vi "Sending Single U32 CMD and String Data.vi"(0 "TCP Ref In":refnum<k5>, 1 "Time Out(ms)":i32=100, 5 "CMD":u32, 9 "Data":string, 11 "error in (no error)":errorcluster) -> (4 "TCP Ref Out":refnum<k5>, 15 "error out":errorcluster)   [LabVIEW 2024]
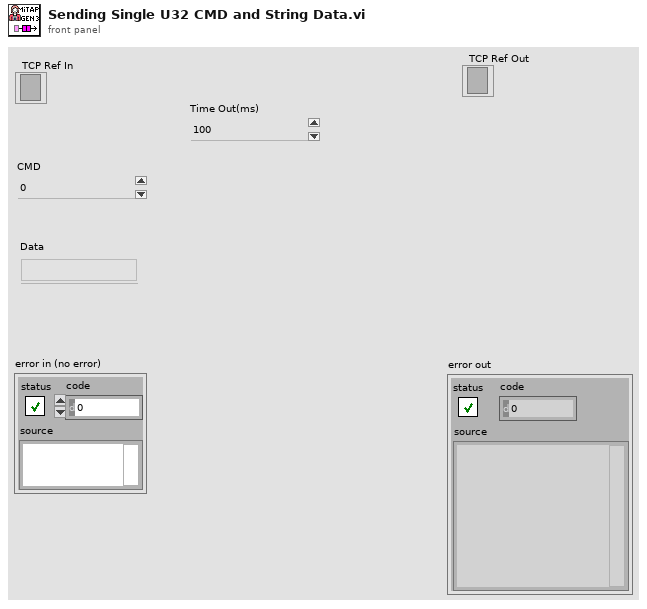
[diagram p1: front panel]
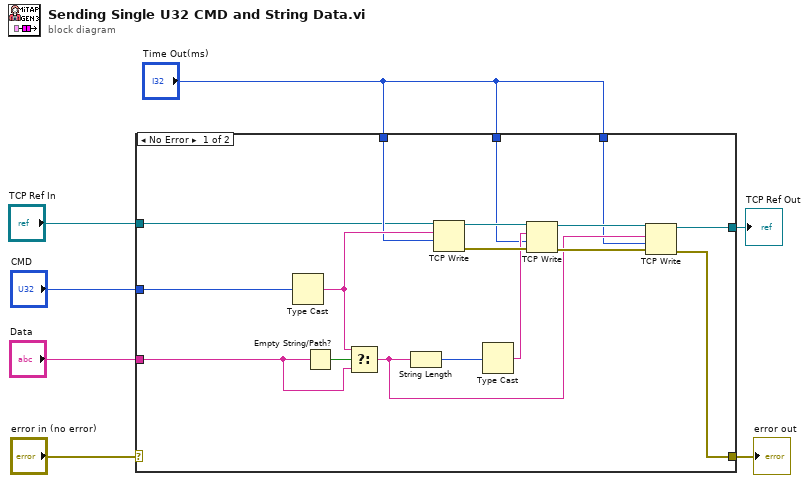
[diagram p0: block diagram]
diagram:
  n1 = case shown="No Error" "error in (no error)" {
    selector: "error in (no error)" -> [_ w25]
    tunnel: [w15 w25] -> w6
    tunnel: "Data" -> [w16 _]
    tunnel: "CMD" -> [w9 _]
    tunnel: "Time Out(ms)" -> [w14 _]
    tunnel: "Time Out(ms)" -> [w13 _]
    tunnel: "Time Out(ms)" -> [w12 _]
    tunnel: "TCP Ref In" -> [w11 _]
    tunnel: [w10 _] -> w1
    frame No Error {
      n2 = Type Cast(x=w9) -> (*(type *) &x=w18:string)  [unwired: 1 in]
      n3 = Empty String/Path?(string/path=w16) -> (empty?=w19:bool)
      n4 = Select(t=w18, s=w19, f=w16) -> (s? t:f=w17:string)
      n5 = String Length(string=w17) -> (length=w8:i32)
      n6 = TCP Write(connection ID=w11, data in=w18, 9:w14) -> (connection ID out=w24:refnum<k5>, error out=w23:errorcluster)  [unwired: 1 in, 1 out]
      n7 = Type Cast(x=w8) -> (*(type *) &x=w20:string)  [unwired: 1 in]
      n8 = TCP Write(connection ID=w24, data in=w20, error in (no error)=w23, 9:w13) -> (connection ID out=w21:refnum<k5>, error out=w22:errorcluster)  [unwired: 1 out]
      n9 = TCP Write(connection ID=w21, data in=w17, error in (no error)=w22, 9:w12) -> (connection ID out=w10:refnum<k5>, error out=w15:errorcluster)  [unwired: 1 out]
    }
    frame Error {
    }
  }
  "error out" <- w6
  "TCP Ref Out" <- w1
